vi "Read Number of Tatics.vi"(8 "error in (no error)":errorcluster, 11 "SimplePassReceiverRole in":refnum<class "SimplePassReceiverRole.lvclass">) -> (0 "error out":errorcluster, 2 "Number of Tatics":dbl, 3 "SimplePassReceiverRole out":refnum<class "SimplePassReceiverRole.lvclass">)   [LabVIEW 2023, in "SimplePassReceiverRole.lvclass"]
uses:
  SimplePassReceiverRole.lvclass
  SimplePassReceiverRole.lvclass/SimplePassReceiverRole.ctl
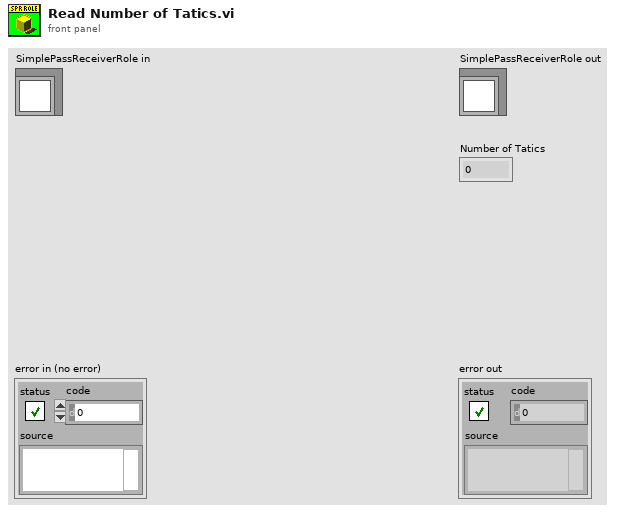
[diagram p1: front panel]
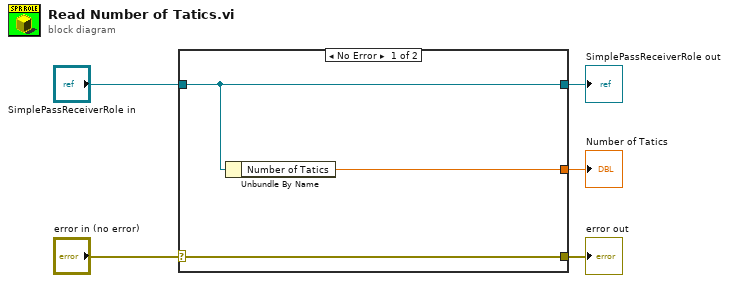
[diagram p0: block diagram]
diagram:
  n1 = case shown="No Error" "error in (no error)" {
    selector: "error in (no error)" -> [w8 w9]
    tunnel: [w8 w9] -> w4
    tunnel: [w7 w10] -> w2
    tunnel: "SimplePassReceiverRole in" -> [w7 w10]
    tunnel: [w6 _] -> w1
    frame No Error {
      n2 = Unbundle By Name(w7) -> ("Number of Tatics"=w6:dbl)
    }
    frame Error {
    }
  }
  "error out" <- w4
  "SimplePassReceiverRole out" <- w2
  "Number of Tatics" <- w1
